vi "get.Field.As.Variant.vi"(8 "error in (no error)":errorcluster, 10 "Field.Name":string, 11 "PitchMessage in":refnum<class "PitchMessage.lvclass">) -> (0 "error out":errorcluster, 2 "Value.Variant":T1, 3 "PitchMessage out":refnum<class "PitchMessage.lvclass">)   [LabVIEW 2022 SP3, in "PitchMessage.lvclass"]
uses:
  PitchMessage.lvclass
  FieldValue.ctl
  PitchMessage.lvclass/PitchMessage.ctl
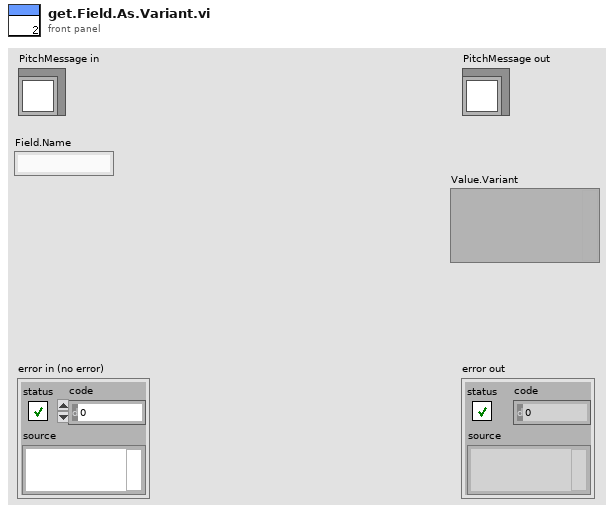
[diagram p1: front panel]
types:
  T1 = typedef "FieldValue.ctl" = variant
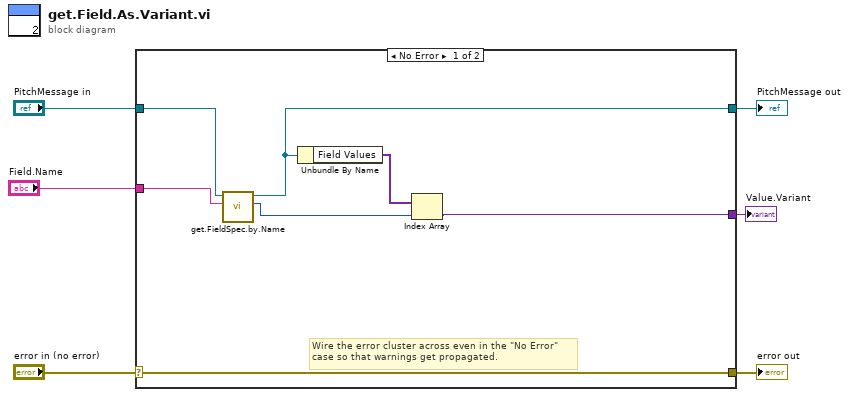
[diagram p0: block diagram]
diagram:
  n1 = case shown="No Error" "error in (no error)" {
    selector: "error in (no error)" -> [w13 w15]
    tunnel: [w13 w15] -> w5
    tunnel: [w8 w14] -> w3
    tunnel: "PitchMessage in" -> [w11 w14]
    tunnel: "Field.Name" -> [w12 _]
    tunnel: [w7 _] -> w1
    frame No Error {
      # "Wire the error cluster across even in the \"No Error\"\ncase so that warnings get propagated."
      n2 = call-dynamic "get.FieldSpec.by.Name.vi"("Field.Name"=w12, "PitchMessage in"=w11) -> ("Index"=w9:i32, "PitchMessage out"=w8:refnum<class "PitchMessage.lvclass">)  [unwired: 7 in, 1 out]
      n3 = Unbundle By Name(w8) -> ("Field Values"=w10:T1[])
      n4 = Index Array(array=w10, index=w9) -> (element=w7:T1)
    }
    frame Error {
    }
  }
  "error out" <- w5
  "PitchMessage out" <- w3
  "Value.Variant" <- w1
